vi "Triggered Continuous Buffered Acquisition with Logging.vi"() -> ()   [LabVIEW 2009]
uses:
  <vilib>/DAQmx/configure/trigger.llb/DAQmx Start Trigger (Digital Edge).vi
  <vilib>/DAQmx/configure/timing.llb/DAQmx Timing (Sample Clock).vi
  <vilib>/DAQmx/create/channels.llb/DAQmx Create Channel (AI-Voltage-Basic).vi
  <vilib>/DAQmx/read.llb/DAQmx Read (Analog Wfm 1Chan NSamp).vi
panel:
  in  "trigger source":tag="/Dev1/PFI1"
  in  "physical channels":tag="Dev1/ai1"
  in  "rate":dbl=1000.0 format="%0.2f"
  in  "stop":bool
  out "data":waveform(dbl)(graph)
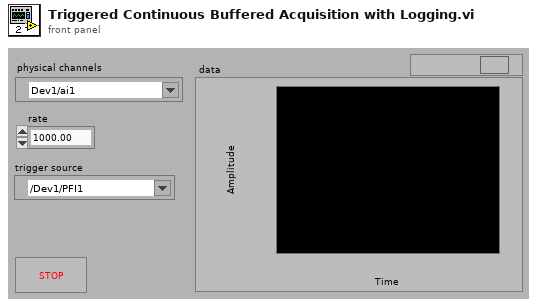
[diagram p1: front panel]
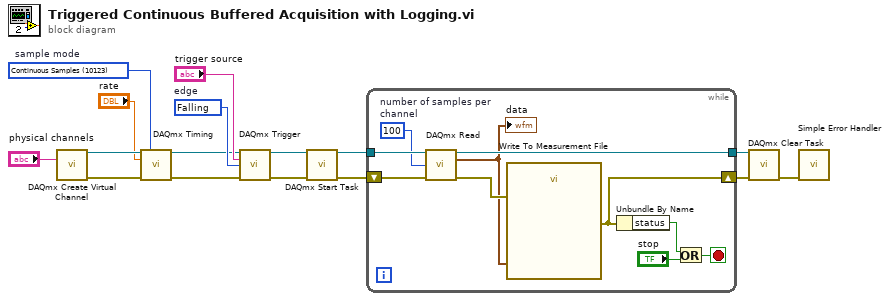
[diagram p0: block diagram]
diagram:
  w15 = 10171 items=["Rising"=10280, "Falling"=10171]  # edge
  w5 = 10123 items=["Finite Samples"=10178, "Continuous Samples"=10123, "Hardware Timed Single Point"=12522]  # sample mode
  n1 = call-poly <vilib>:"DAQmx Create Virtual Channel.vi"("physical channels"="physical channels") -> ("task out"=w14:refnum<k21>, "error out"=w13:errorcluster)  [unwired: 13 in]
  n2 = call-poly <vilib>:"DAQmx Timing.vi"("task/channels in"=w14, "sample mode"=w5, "rate"="rate", "error in"=w13) -> ("task out"=w7:refnum<k21>, "error out"=w6:errorcluster)  [unwired: 10 in]
  n3 = call-poly <vilib>:"DAQmx Trigger.vi"("task/channels in"=w7, "source"="trigger source", "edge"=w15, "error in"=w6) -> ("task out"=w12:refnum<k21>, "error out"=w10:errorcluster)  [unwired: 10 in]
  n4 = call <vilib>:"DAQmx Start Task.vi"("task/channels in"=w12, "error in"=w10) -> ("task out"=w11:refnum<k21>, "error out"=w9:errorcluster)  [unwired: 12 in]
  n5 = while {
    tunnel: [w21] -> w1
    tunnel: w11 -> [w25]
    shift-right: [w19] -> w2
    shift-left: w9 -> [w26]
    stop <- w24 stop-if-true
    w17 = 100  # number of samples per channel
    n6 = call-poly <vilib>:"DAQmx Read.vi"("task/channels in"=w25, "number of samples per channel"=w17, "error in"=w26) -> ("task out"=w21:refnum<k21>, "data"=w18:waveform(dbl), "error out"=w20:errorcluster)  [unwired: 10 in]
    "data" <- w18
    n7 = call "Write To Measurement File"("Signals"=w18, "error in (no error)"=w20) -> ("error out"=w19:errorcluster)  [unwired: 15 in, 2 out]
    n8 = Unbundle By Name "Unbundle By Name"(w19) -> ("status"=w22:bool)
    n9 = Or(x=w22, y="stop") -> (x .or. y?=w24:bool)
  }
  n10 = call <vilib>:"DAQmx Clear Task.vi"("task in"=w1, "error in"=w2) -> ("error out"=w3:errorcluster)  [unwired: 13 in]
  n11 = call <vilib>:"Simple Error Handler.vi"("error in (no error)"=w3) -> ()  [unwired: 4 in, 5 out]
